vi "setUp.vi"(8 "error in":errorcluster, 11 "reference in":refnum<class "Embedded Data Logger Common System Tests.lvclass">) -> (0 "error out":errorcluster, 3 "reference out":refnum<class "Embedded Data Logger Common System Tests.lvclass">)   [LabVIEW 2027, in "Embedded Data Logger Common System Tests.lvclass"]
doc: "setUp runs prior to the test method during test execution. Use this method to initialize any object data required by your tests."
uses:
  Embedded Data Logger Common System Tests.lvclass
  <vilib>/addons/_JKI Toolkits/VI Tester/TestCase.llb/TestCase.lvclass
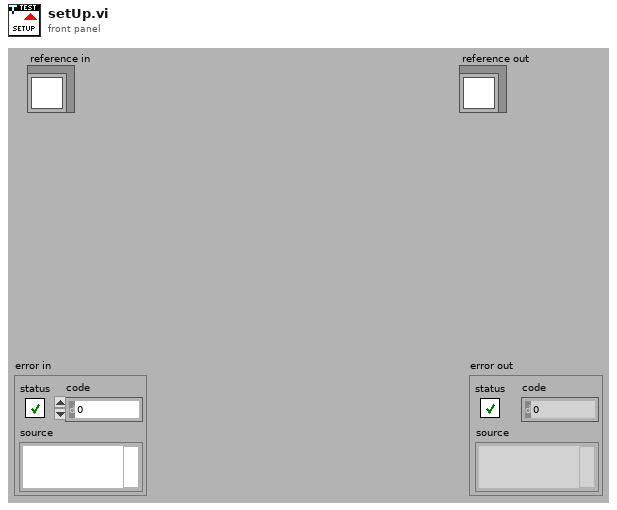
[diagram p1: front panel]
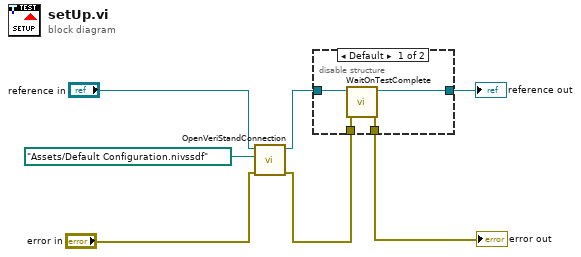
[diagram p0: block diagram]
diagram:
  n1 = call-dynamic "OpenVeriStandConnection.vi"("error in (no error)"="error in", "System Definition File"=path "Assets/Default Configuration.nivssdf", "VeriStand Test Case in"="reference in") -> ("error out"=w4:errorcluster, "VeriStand Test Case out"=w3:refnum<class "Embedded Data Logger Common System Tests.lvclass">)  [unwired: 6 in, 1 out]
  n2 = disable-structure shown="Default" {
    disable-tunnel: w4 -> [w11 w12]
    disable-tunnel: [w10 w12] -> w7
    disable-tunnel: [w9 w13] -> w6
    disable-tunnel: w3 -> [w8 w13]
    frame condition #0 (active) {
      n3 = call <vilib>:"WaitOnTestComplete.vi"("error in (no error)"=w11, "TestCase in"=w8) -> ("error out"=w10:errorcluster, "TestCase out"=w9:refnum<class "Embedded Data Logger Common System Tests.lvclass">)  [unwired: 8 in]
    }
    frame condition #1 {
    }
  }
  "error out" <- w7
  "reference out" <- w6
